vi "Read connect timeout.vi"(8 "error in (no error)":errorcluster, 11 "VISA TCP in":refnum<class "VISA TCP.lvclass">) -> (0 "error out":errorcluster, 2 "connect timeout":i32=10000, 3 "VISA TCP out":refnum<class "VISA TCP.lvclass">)   [LabVIEW 2021, in "Sockets.lvlib" / "VISA TCP.lvclass"]
uses:
  VISA TCP.lvclass/VISA TCP.ctl
  VISA TCP.lvclass
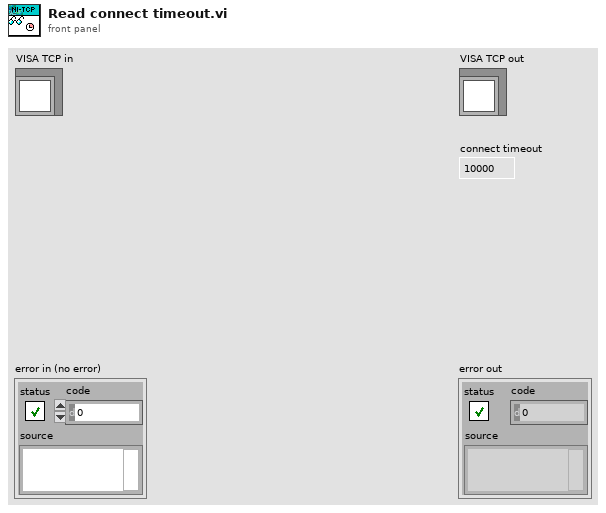
[diagram p1: front panel]
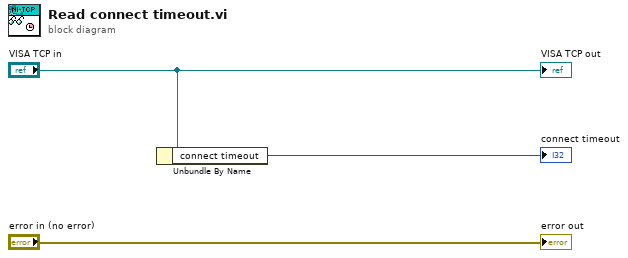
[diagram p0: block diagram]
diagram:
  n1 = Unbundle By Name("VISA TCP in") -> ("connect timeout"=→"connect timeout":i32)
  "error out" <- "error in (no error)"
  "VISA TCP out" <- "VISA TCP in"
